vi "Add User.vi"(6 "New Password":string, 7 "New User":string, 8 "error in (no error)":errorcluster, 9 "Confirm Password":string, 10 "Work Group":string, 11 "Refnum in":T1) -> (0 "error out":errorcluster)   [LabVIEW 2018]
uses:
  <vilib>/addons/database/Connection.llb/Conn ObjectReference.ctl
  <vilib>/addons/database/Connection.llb/Conn Execute.vi
  <vilib>/addons/database/Recordset.llb/Rec Destroy - Connection.vi
  <vilib>/addons/database/NI_Database_API.lvlib
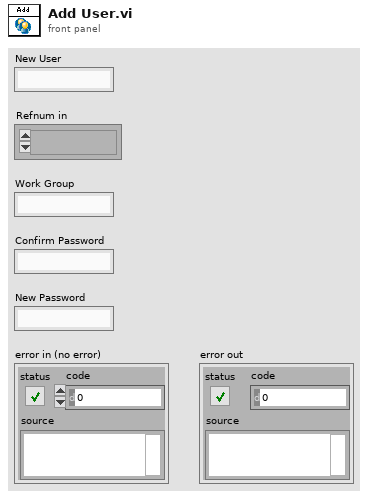
[diagram p1: front panel]
types:
  T1 = typedef "NI_Database_API.lvlib/Conn ObjectReference.ctl" = refnum<k1>
  T2 = typedef "NI_Database_API.lvlib/Rec ObjectReference.ctl" = refnum<k1>
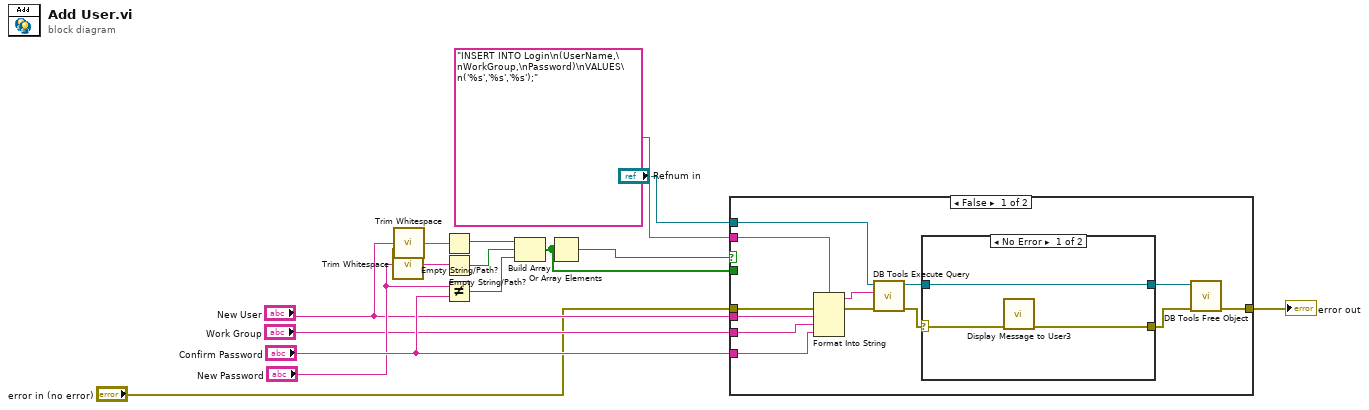
[diagram p0: block diagram]
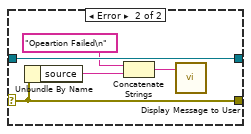
[diagram p2: hidden frame]
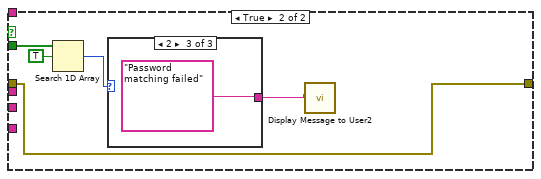
[diagram p3: hidden frame]
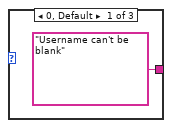
[diagram p4: hidden frame]
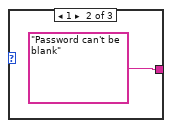
[diagram p5: hidden frame]
diagram:
  n1 = call <vilib>:"Trim Whitespace.vi"("string"="New Password") -> ("trimmed string"=w8:string)  [unwired: 1 in]
  n2 = call <vilib>:"Trim Whitespace.vi"("string"="New User") -> ("trimmed string"=w7:string)  [unwired: 1 in]
  n3 = Empty String/Path?(string/path=w7) -> (empty?=w9:bool)
  n4 = Empty String/Path?(string/path=w8) -> (empty?=w10:bool)
  n5 = Not Equal?(x="New Password", y="Confirm Password") -> (x != y?=w13:bool)
  n6 = Build Array(w9, w10, w13) -> (w15:bool[])
  n7 = Or Array Elements(Boolean array=w15) -> (logical OR=w14:bool)
  n8 = case shown="False" w14 {
    tunnel: [w28 w38] -> w1
    tunnel: "Refnum in" -> [w27 _]
    tunnel: "INSERT INTO Login\n(UserName,\nWorkGroup,\nPassword)\nVALUES\n('%s','%s','%s');" -> [w26 _]
    tunnel: "error in (no error)" -> [w24 w38]
    tunnel: "Work Group" -> [w22 _]
    tunnel: "New User" -> [w21 _]
    tunnel: "Confirm Password" -> [w20 _]
    tunnel: w15 -> [_ w41]
    frame False {
      n9 = Format Into String(format string=w26, error in=w24, w21, w22, w20) -> (resulting string=w25:string, error out=w23:errorcluster)  [unwired: 1 in]
      n10 = call-poly <vilib>:"DB Tools Execute Query.vi"("error in (no error)"=w23, "SQL query"=w25, "connection reference"=w27) -> ("error out"=w19:errorcluster, "recordset reference"=w17:T2)  [unwired: 5 in]
      n11 = case shown="No Error" w19 {
        selector: w19 -> [w30 w35]
        tunnel: [w29 w35] -> w18
        tunnel: w17 -> [w31 w36]
        tunnel: [w31 w36] -> w16
        frame No Error {
          n12 = call "Display Message to User3"("error in (no error)"=w30) -> ("error out"=w29:errorcluster)  [unwired: 9 in, 1 out]
        }
        frame Error {
          n13 = Unbundle By Name(w35) -> ("source"=w34:string)
          n14 = Concatenate Strings("Opeartion Failed\n" ("string"), w34) -> (w33:string)
          n15 = call "Display Message to User"("Message"=w33) -> ()  [unwired: 9 in, 2 out]
        }
      }
      n16 = call-poly <vilib>:"DB Tools Free Object.vi"("error in (no error)"=w18, "recordset reference"=w16) -> ("error out"=w28:errorcluster)  [unwired: 8 in, 1 out]
    }
    frame True {
      n17 = Search 1D Array(1D array=w41, element=TRUE) -> (index of element=w39:i32)  [unwired: 1 in]
      n18 = case shown="2" w39 {
        tunnel: ["Username can't be blank" "Password can't be blank" "Password matching failed"] -> w37
        frame 0, Default {
        }
        frame 1 {
        }
        frame 2 {
        }
      }
      n19 = call "Display Message to User2"("Message"=w37) -> ()  [unwired: 9 in, 2 out]
    }
  }
  "error out" <- w1
